vi "Initialize Do.vi"(8 "error in (no error)":errorcluster, 11 "Instrument in":refnum<class "DMM.NI.Simulate.lvclass">) -> (0 "error out":errorcluster, 3 "Instrument out":refnum<class "DMM.NI.Simulate.lvclass">)   [LabVIEW 2020, in "NI DMM Driver.lvlib" / "DMM.NI.Simulate.lvclass"]
doc: "Initialize the Instrument.\n\nInitialize a simulated NI DMM with the contained Alias. If the contained Alias is empty the alias SimulatedDMM is used."
uses:
  DMM.NI.Simulate.lvclass
  C:/Current Projects/WS/LV32.2020.HDH.Driver.DMM/DMM.NI/NI/DMM.NI.lvclass
  NI/DMM.NI.lvclass/DMM.NI.ctl
  NI/DMM.NI.lvclass
  C:/Current Projects/WS/PPL/HDH.Actor Framework.Core.Instrument Driver.lvlibp/Instrument Driver/Instrument Driver.lvclass
  PPL/HDH.Actor Framework.Core.Instrument Driver.lvlibp/Instrument Driver/Instrument Driver.lvclass
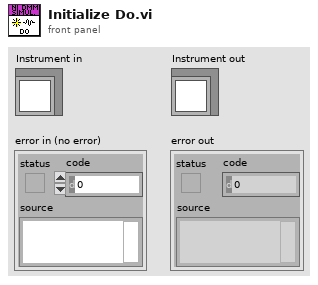
[diagram p1: front panel]
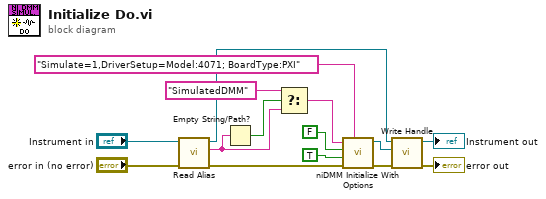
[diagram p0: block diagram]
diagram:
  n1 = call "Read Alias.vi"("error in (no error)"="error in (no error)", "Instrument in"="Instrument in") -> ("error out"=w11:errorcluster, "Alias"=w3:string, "Instrument out"=w9:refnum<class "DMM.NI.Simulate.lvclass">)  [unwired: 7 in]
  n2 = Empty String/Path?(string/path=w3) -> (empty?=w4:bool)
  n3 = Select(t="SimulatedDMM", s=w4, f=w3) -> (s? t:f=w1:string)
  n4 = call <instrlib>:"niDMM Initialize With Options.vi"("Option String"="Simulate=1,DriverSetup=Model:4071; BoardType:PXI", "error in (no error)"=w11, "Reset Device"=TRUE, "ID Query"=FALSE, "Instrument Descriptor"=w1) -> ("error out"=w7:errorcluster, "instrument handle out"=w10:refnum<k15>)  [unwired: 5 in]
  n5 = call "Write Handle.vi"("error in (no error)"=w7, "NI DMM"=w10, "NI DMM Driver in"=w9) -> ("error out"=→"error out":errorcluster, "NI DMM Driver out"=→"Instrument out":refnum<class "DMM.NI.Simulate.lvclass">)  [unwired: 7 in]
